vi "Matrix Mult and show result.vi"() -> ()   [LabVIEW 2014, in "Arduino MatrixMath.lvlib"]
uses:
  Arduino MatrixMath.lvlib
  <vilib>/LabVIEW Universal Transcriptor/LabVIEW for Arduino SoftwareSerial Library/Arduino SoftwareSerial Wrapper.lvlib
panel:
  in  "A":sgl[](array[numeric])=[1.0, 2.0, 3.0, 4.0, 5.0, 6.0, 7.0, 8.0]
  in  "B":sgl[](array[numeric])=[1.0, 2.0, 3.0, 4.0, 5.0, 6.0, 7.0, 8.0]
  out "Error Out":errorcluster
  in  "Error In":errorcluster
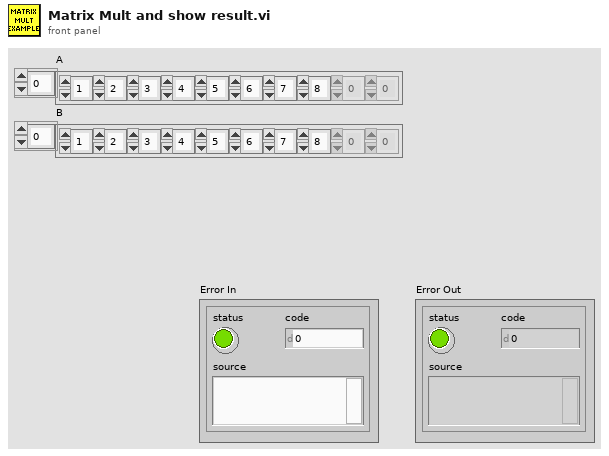
[diagram p1: front panel]
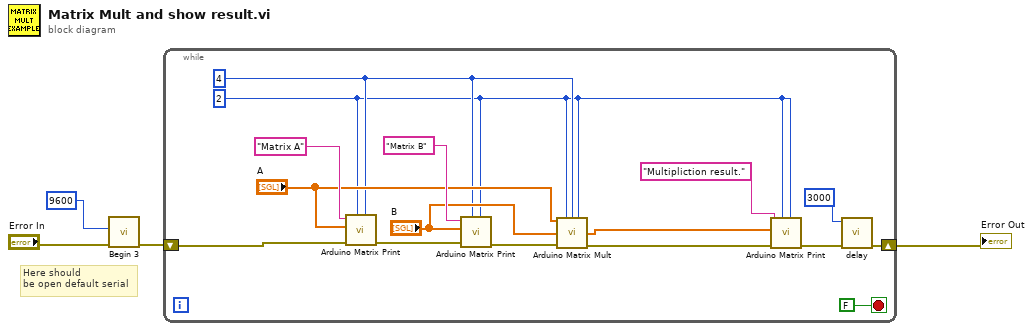
[diagram p0: block diagram]
diagram:
  # "Here should\nbe open default serial"
  n1 = call <vilib>:"Begin 3.vi"("Error In"="Error In", "Baudrate"=u16 9600 ("Speed")) -> ("Error Out"=w3:errorcluster)  [unwired: 8 in]
  n2 = while {
    shift-right: [w7] -> w4
    shift-left: w3 -> [w19]
    stop <- FALSE stop-if-true
    w10 = u8 4 ("cols num.")
    w8 = u8 2 ("rows num.")
    n3 = call "Arduino Matrix Print.vi"("cols num."=w10, "rows num."=w8, "Error In"=w19, "A"="A", "Label"="Matrix A") -> ("Error Out"=w16:errorcluster)  [unwired: 6 in]
    n4 = call "Arduino Matrix Print.vi"("cols num."=w8, "rows num."=w10, "Error In"=w16, "A"="B", "Label"="Matrix B") -> ("Error Out"=w14:errorcluster)  [unwired: 6 in]
    n5 = call "Arduino Matrix Mult.vi"("A"="A", "A rows"=w8, "A cols = B rows"=w10, "B cols"=w8, "B"="B", "Error In"=w14) -> ("A*B"=w9:sgl[], "Error Out"=w13:errorcluster)  [unwired: 8 in]
    n6 = call "Arduino Matrix Print.vi"("cols num."=w8, "rows num."=w8, "Error In"=w13, "A"=w9, "Label"="Multipliction result.") -> ("Error Out"=w6:errorcluster)  [unwired: 6 in]
    n7 = call <vilib>:"delay.vi"("Error In"=w6, "time (ms)"=3000) -> ("Error Out"=w7:errorcluster)  [unwired: 9 in]
  }
  "Error Out" <- w4
